vi "Untitled 1 (SubVI).vi"(11 "Buttons[1]":bool) -> ()   [LabVIEW 2015]
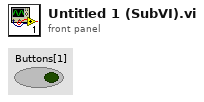
[diagram p1: front panel]
types:
  T1 = typedef "WPI_PotentiometerDevRef.ctl" = cluster{"DevStatus":errorcluster, "Analog Channel":T2, "Invert Output":bool}
  T2 = typedef "FPGA_AIChannel.ctl" = enum8{"AI 0", "AI 1", "AI 2", "AI 3", "AI MXP 0", "AI MXP 1", "AI MXP 2", "AI MXP 3", "Invalid"}
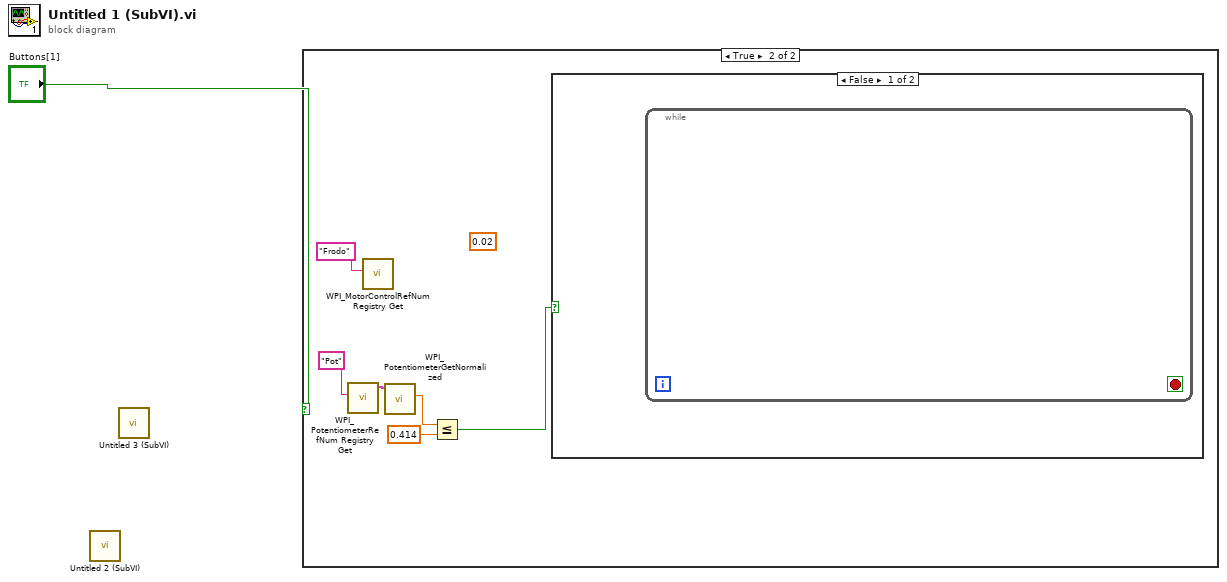
[diagram p0: block diagram]
diagram:
  n1 = call "Untitled 2 (SubVI).vi"() -> ()  [unwired: 12 in]
  n2 = call "Untitled 3 (SubVI).vi"() -> ()  [unwired: 12 in]
  n3 = case shown="True" "Buttons[1]" {
    frame False {
    }
    frame True {
      (unwired) 0.02
      n4 = call <vilib>:"WPI_PotentiometerRefNum Registry Get.vi"("refnum name"="Pot") -> ("PotDevRef"=w6:T1)  [unwired: 9 in, 1 out]
      n5 = call <vilib>:"WPI_MotorControlRefNum Registry Get.vi"("refnum name"="Frodo") -> ()  [unwired: 9 in, 2 out]
      n6 = call <vilib>:"WPI_PotentiometerGetNormalized.vi"("PotDevRef"=w6) -> ("Normalized Value"=w5:dbl)  [unwired: 8 in, 2 out]
      n7 = Less Or Equal?(x=w5, y=0.414) -> (x <= y?=w3:bool)
      n8 = case shown="False" w3 {
        frame False {
          n9 = while {
            stop <- _ stop-if-true
          }
        }
        frame True {
          n10 = while {
            stop <- _ stop-if-true
          }
        }
      }
    }
  }
